vi "周期设置.vi"(11 "定时控制参数输入":T1) -> (3 "定时控制参数输出":T1)   [LabVIEW 2016, in "斯坦道氨氮.lvlib"]
panel:
  in  "确定":bool
  in  "取消":bool
  in  "定时功能启用":bool
  out "选项卡控件":enum32{"定点启动", "间隔启动"}(tab)
  in  "24H周期设置":bool[](xcontrol)
  in  "定时间隔":dbl
  in  "周期设置类型":enum16{"定点启动", "间隔启动"}(ring)
  in  "仪器测试类型":enum16{"水样测试", "标样核查", "空白测试", "跨度核查"}(ring)
  # "仪器测试类型："
  # "周期设置类型："
  # "请输入定时启动间隔"
  # "min"
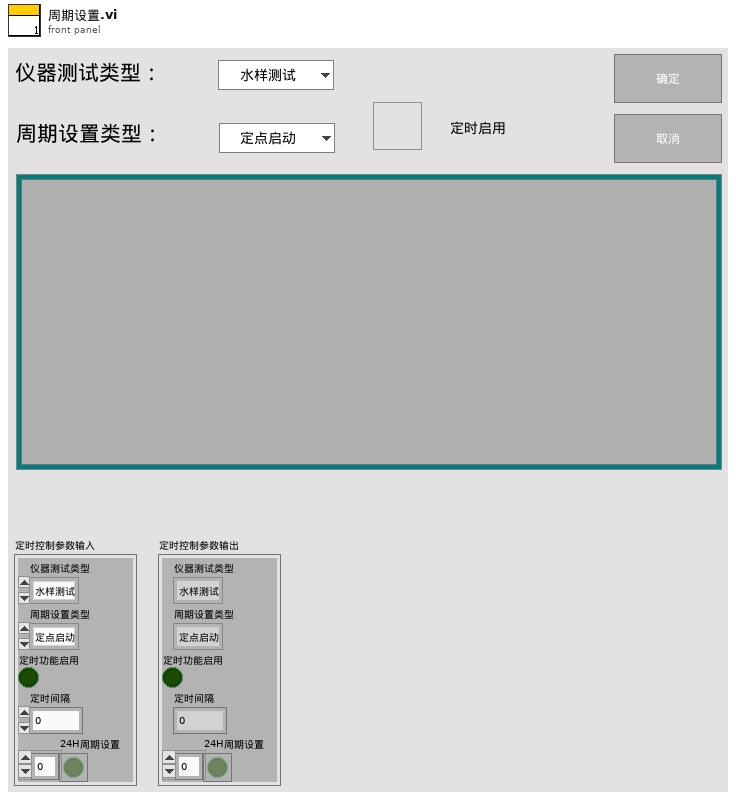
[diagram p1: front panel]
types:
  T1 = cluster{"仪器测试类型":enum16{"水样测试", "标样核查", "空白测试", "跨度核查"}, "周期设置类型":enum16{"定点启动", "间隔启动"}, "定时功能启用":bool, "定时间隔":dbl, "24H周期设置":bool[]}
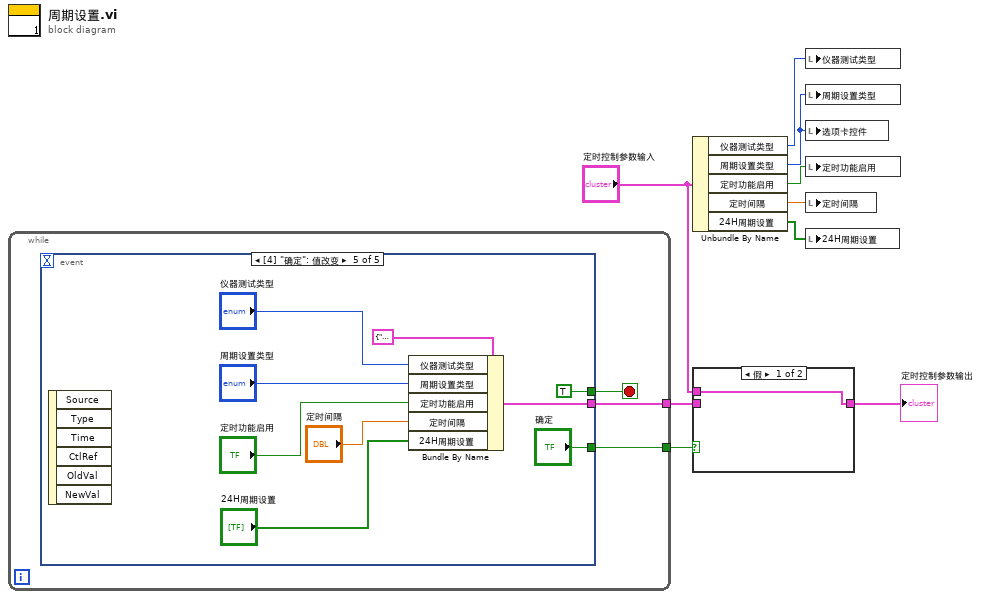
[diagram p0: block diagram]
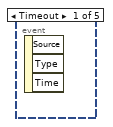
[diagram p3: hidden frame]
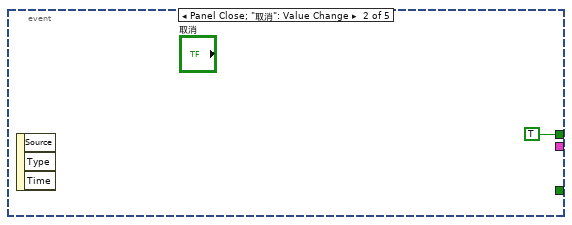
[diagram p4: hidden frame]
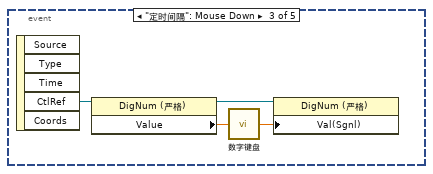
[diagram p5: hidden frame]
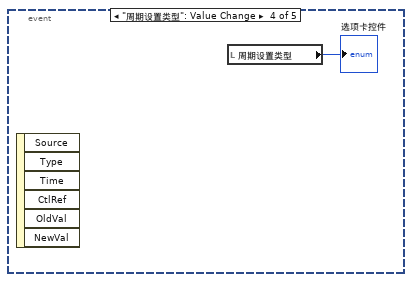
[diagram p6: hidden frame]
diagram:
  n1 = while {
    tunnel: [w11] -> w3
    tunnel: [w10] -> w4
    stop <- w12 stop-if-true
    n2 = event shown="[4] \"确定\": 值改变" {
      selector: _ -> [_ _ _ _ _]
      dyn-events: _ -> [_ _ _ _ _]
      timeout: _ -> [_ _ _ _ _]
      tunnel: [_ TRUE _ _ TRUE] -> w12
      tunnel: [_ _ _ _ w21] -> w11
      tunnel: [_ _ _ _ "确定"] -> w10
      event Timeout {
        n3 = event-data() -> ()  [unwired: 1 in, 3 out]
      }
      event Panel Close; "取消": Value Change {
        n4 = event-data() -> ()  [unwired: 1 in, 3 out]
      }
      event "定时间隔": Mouse Down {
        n5 = event-data() -> ("CtlRef"=w17:refnum<vi>)  [unwired: 1 in, 4 out]
        n6 = property class="DigNum (严格)"(reference=w17) -> (reference out=w14:refnum<vi>, "Value"=w16:dbl)  [unwired: 1 in, 1 out]
        n7 = call "数字键盘.vi"("OldNumber"=w16) -> ("NewNumber"=w15:dbl)
        n8 = property class="DigNum (严格)"(reference=w14, "Val(Sgnl)"=w15) -> ()  [unwired: 1 in, 2 out]
      }
      event "周期设置类型": Value Change {
        n9 = event-data() -> ()  [unwired: 1 in, 6 out]
        n10 = local read "周期设置类型"() -> (→"选项卡控件":enum16{"定点启动", "间隔启动"})
      }
      event "确定": Value Change {
        n11 = event-data() -> ()  [unwired: 1 in, 6 out]
        n12 = Bundle By Name(cluster=T1 {"仪器测试类型"=enum."水样测试", "周期设置类型"=enum."定点启动", "定时功能启用"=FALSE, "定时间隔"=0.0, "24H周期设置"=[]} ("定时控制"), "仪器测试类型"="仪器测试类型", "周期设置类型"="周期设置类型", "定时功能启用"="定时功能启用", "定时间隔"="定时间隔", "24H周期设置"="24H周期设置") -> (w21:T1)
      }
    }
  }
  n13 = Unbundle By Name("定时控制参数输入") -> ("仪器测试类型"=w9:enum16{"水样测试", "标样核查", "空白测试", "跨度核查"}, "周期设置类型"=w5:enum16{"定点启动", "间隔启动"}, "定时功能启用"=w8:bool, "定时间隔"=w7:dbl, "24H周期设置"=w6:bool[])
  n14 = case shown="假" w4 {
    tunnel: w3 -> [_ w29]
    tunnel: [w28 w29] -> w2
    tunnel: "定时控制参数输入" -> [w28 _]
    frame False {
    }
    frame True {
    }
  }
  "定时控制参数输出" <- w2
  n15 = local write "仪器测试类型"(w9) -> ()
  n16 = local write "周期设置类型"(w5) -> ()
  n17 = local write "选项卡控件"(w5) -> ()
  n18 = local write "定时功能启用"(w8) -> ()
  n19 = local write "定时间隔"(w7) -> ()
  n20 = local write "24H周期设置"(w6) -> ()
